vi "CSConnect.ProcCases.vi"(0 "i ref in":refnum<vi>, 1 "selector":string, 2 "Data":T1, 3 "call cluster":T2={"Object"="", "Selector"="", "CallType"=enum."synchronous", "Async Object"="", "Async Selector"="", "Data Descriptor"="", "Data"=[], "Error #"=0, "Expire"=0}, 5 "error in (no error)":errorcluster) -> (14 "i ref out":refnum<vi>, 17 "answer cluster":T2={"Object"="", "Selector"="", "CallType"=enum."synchronous", "Async Object"="", "Async Selector"="", "Data Descriptor"="", "Data"=[], "Error #"=0, "Expire"=0}, 19 "error out":errorcluster)   [LabVIEW 2014, in "CSConnect.lvlib"]
doc: "This method is called by a process from within the default case in the event loop. The methods of a class that are linked to events will be called from THIS method. Add your code here."
uses:
  CSConnect.lvlib
  CSCore/CSSystem/CoreDefs/CoreDefs.call_type.ctl
  CSCore/BaseProcess/BaseProcess.descriptor string definition.ctl
  CSCore/CSSystem/CoreDefs/CoreDefs.rawDataType.ctl
  CSCore/CSApplicationBaseClasses/PSChannelBase/PSChannelBase.directionType.ctl
  CSCore/CSApplicationBaseClasses/PSChannelBase/PSChannelBase.serviceType.ctl
  CSCore/CSSystem/CoreLib/CoreLib.string 2 byte array.vi
  CSCore/CSSystem/CoreLib/CoreLib.double 2 byte array.vi
  CSCore/CSSystem/CoreLib/CoreLib.byte array 2 double.vi
  CSCore/CSSystem/CoreLib/CoreLib.byte array 2 short.vi
  CSCore/CSSystem/CoreLib/CoreLib.byte array 2 int.vi
  CSCore/CSSystem/CoreLib/CoreLib.lvlib
  CSCore/BaseProcess/BaseProcess.lvlib
  CSCore/CSApplicationBaseClasses/PSChannelBase/PSChannelBase.lvlib
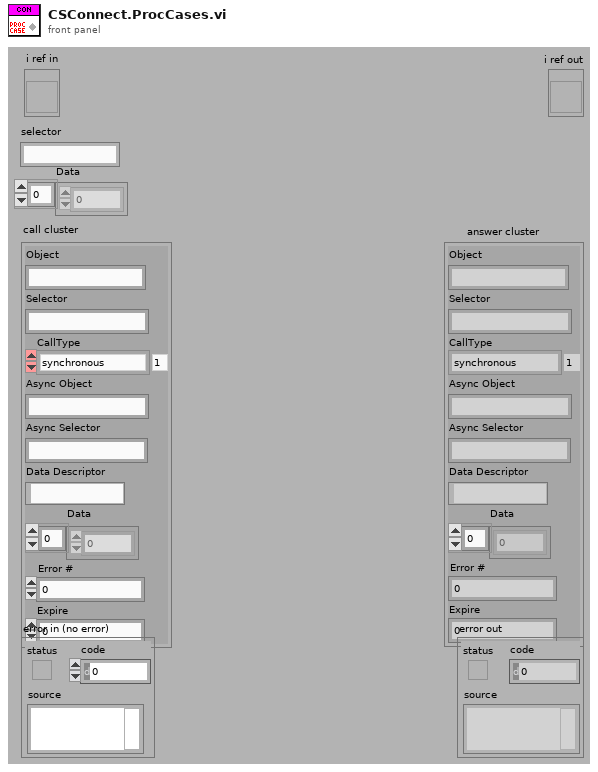
[diagram p1: front panel]
types:
  T1 = typedef "CoreDefs.rawDataType.ctl" = i8[]
  T2 = typedef "CoreDefs.call_type.ctl" = cluster{"Object":string, "Selector":string, "CallType":enum16{"simple", "synchronous", "asynchronous"}, "Async Object":string, "Async Selector":string, "Data Descriptor":T3, "Data":T1, "Error #":i32, "Expire":u32}
  T3 = typedef "BaseProcess.lvlib/BaseProcess.descriptor string definition.ctl" = string
  T4 = typedef "PSChannelBase.lvlib/PSChannelBase.serviceType.ctl" = enum16{"onOff", "voltage", "current", "tripCurrent", "rampUpSpeed", "rampDownSpeed", "status"}
  T5 = typedef "PSChannelBase.lvlib/PSChannelBase.directionType.ctl" = enum16{"unknown", "update actual value", "update nominal value", "update both"}
  T6 = typedef "CSConnect.lvlib/CSConnect.i attribute.ctl" = cluster{"In-Array":cluster{"Alias":string, "Value":dbl, "neededOuts":bool[]}[], "Out-Array":cluster{"ObjectName":string, "VoltFunctionName":string, "OnOffFunctionName":string, "Channel":string, "Calculation-Formula":string}[], "OutChannelsID":i32, "InOutMatrixID":i32}
  T7 = cluster{"ObjectName":string, "VoltFunctionName":string, "OnOffFunctionName":string, "Channel":string, "Calculation-Formula":string}[]
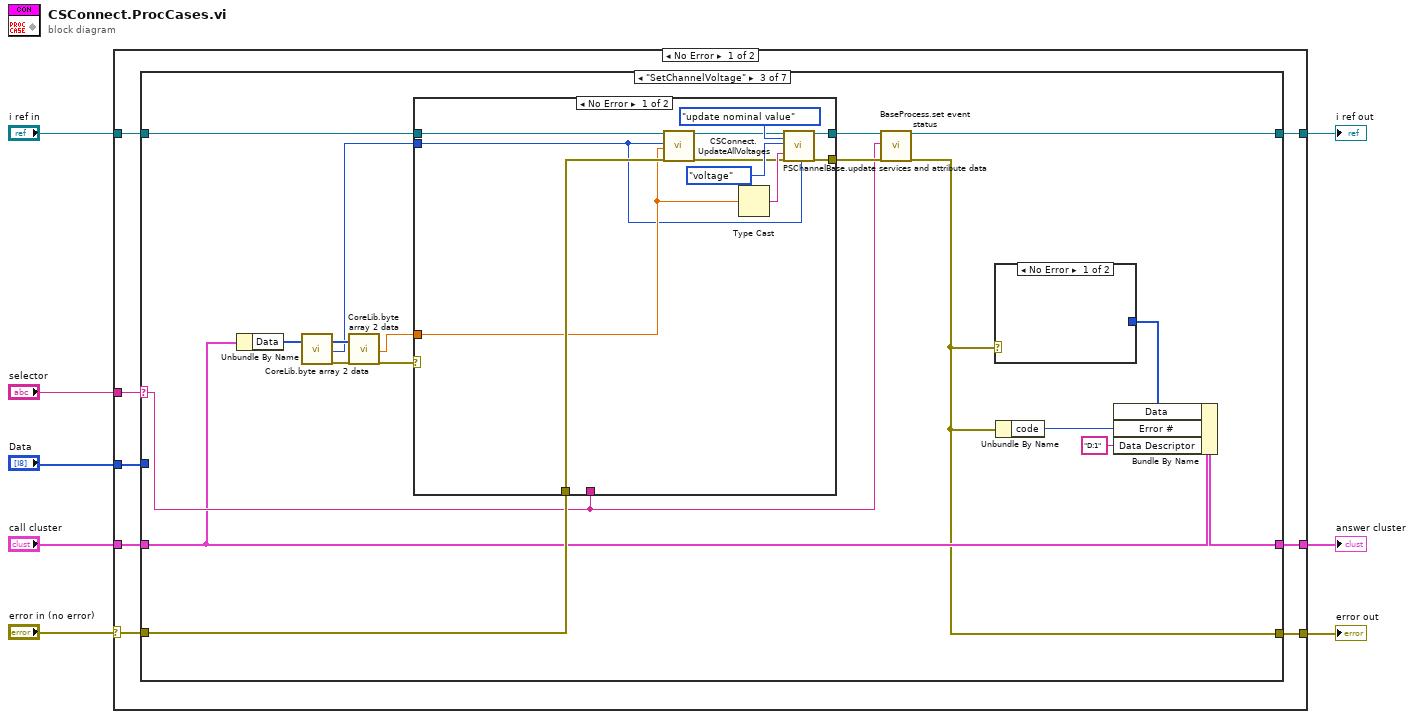
[diagram p0: block diagram]
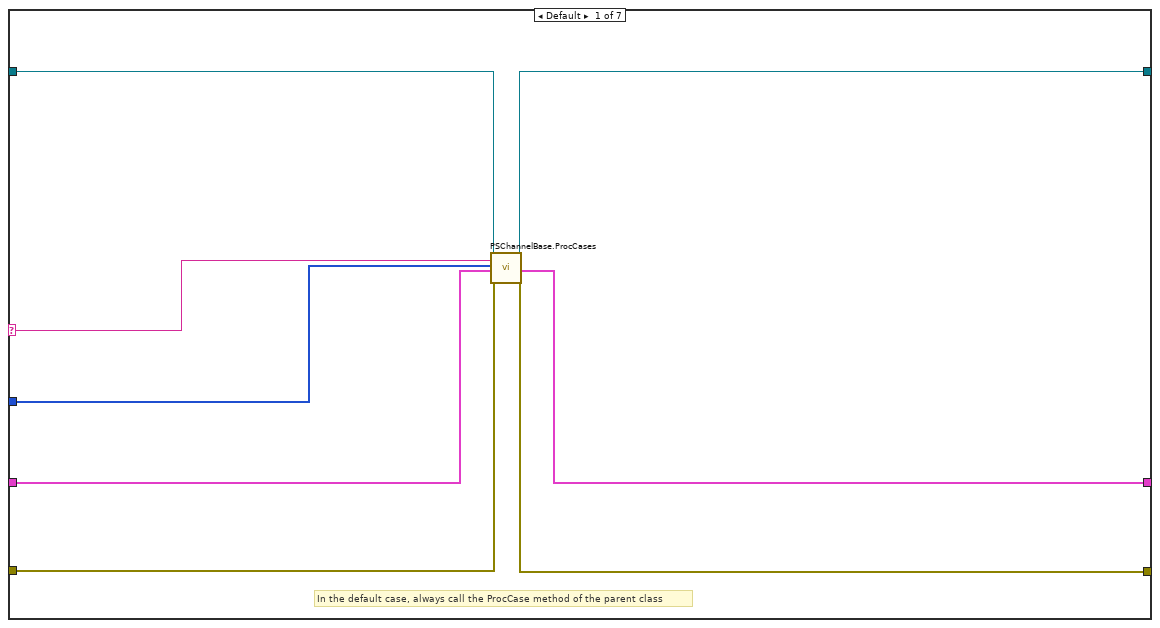
[diagram p2: hidden frame]
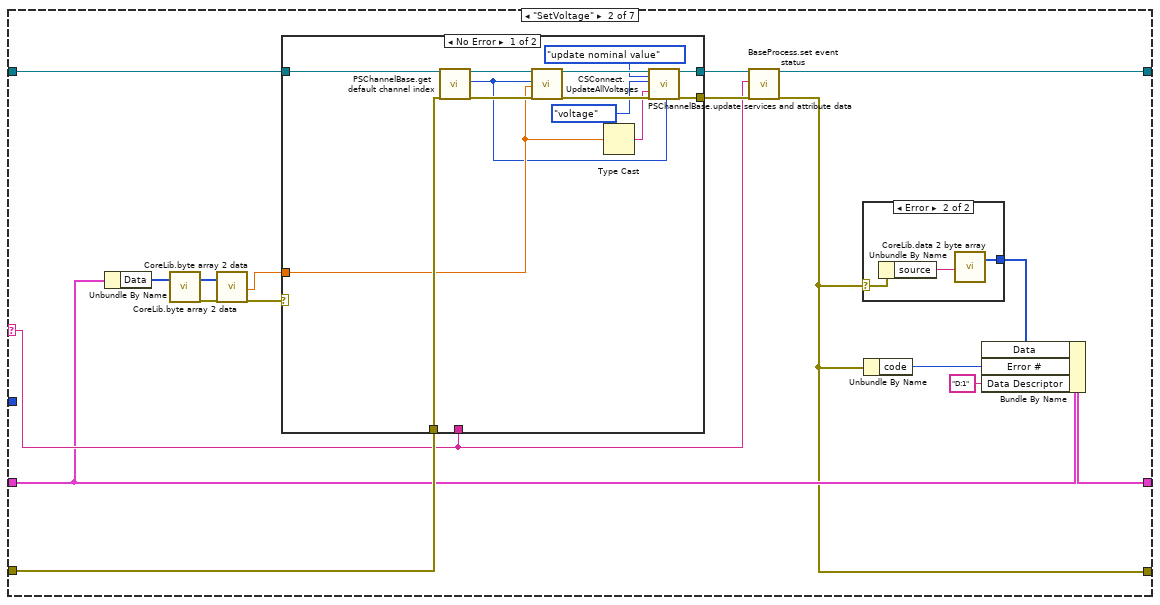
[diagram p3: hidden frame]
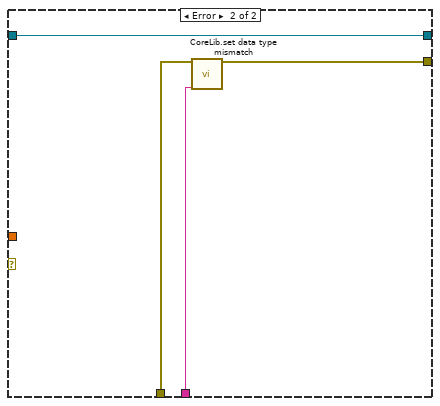
[diagram p5: hidden frame]
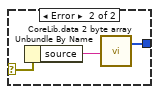
[diagram p6: hidden frame]
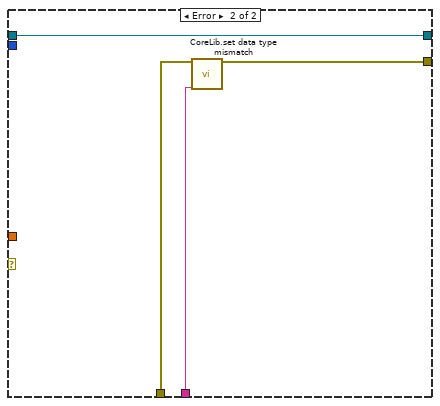
[diagram p7: hidden frame]
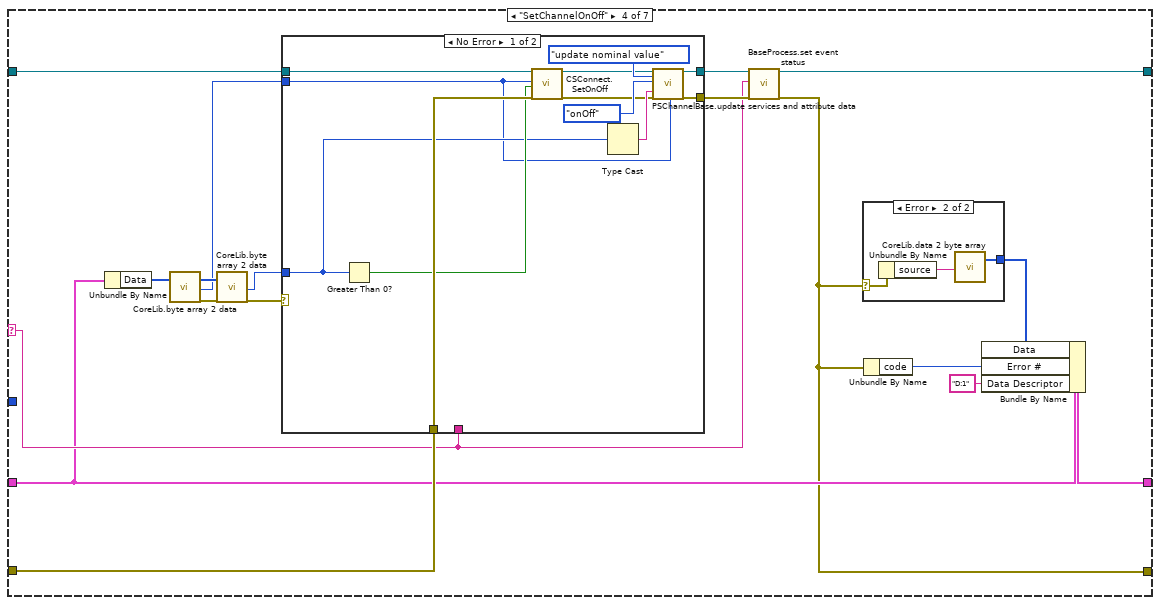
[diagram p8: hidden frame]
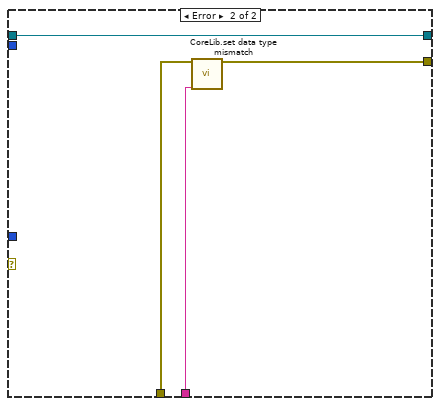
[diagram p10: hidden frame]
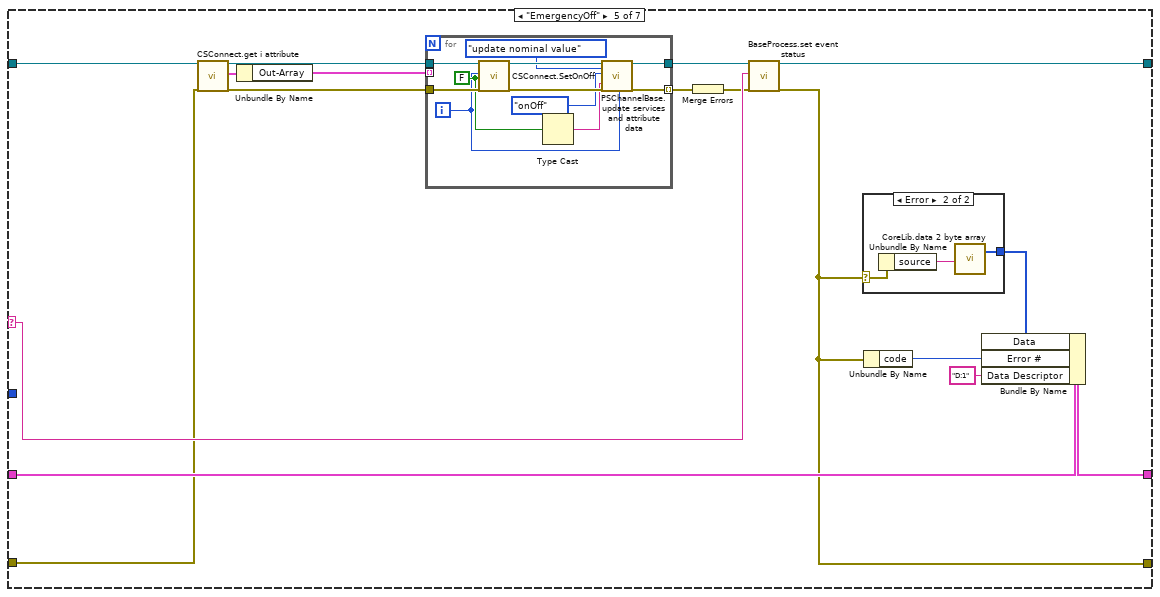
[diagram p11: hidden frame]
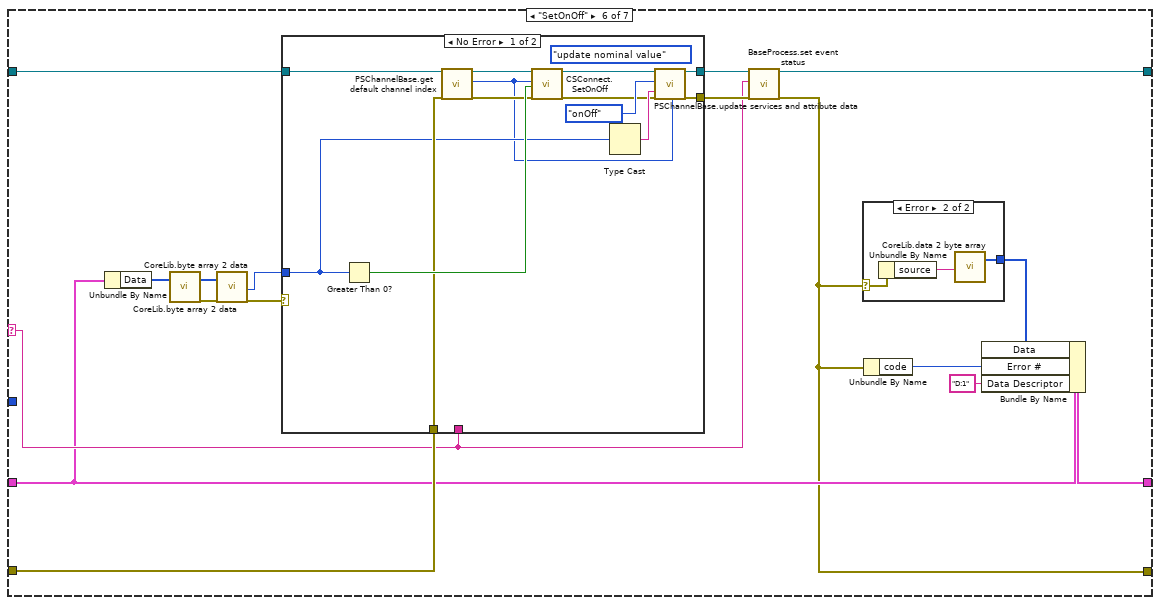
[diagram p13: hidden frame]
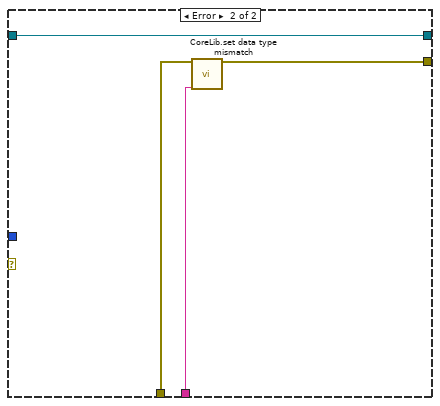
[diagram p15: hidden frame]
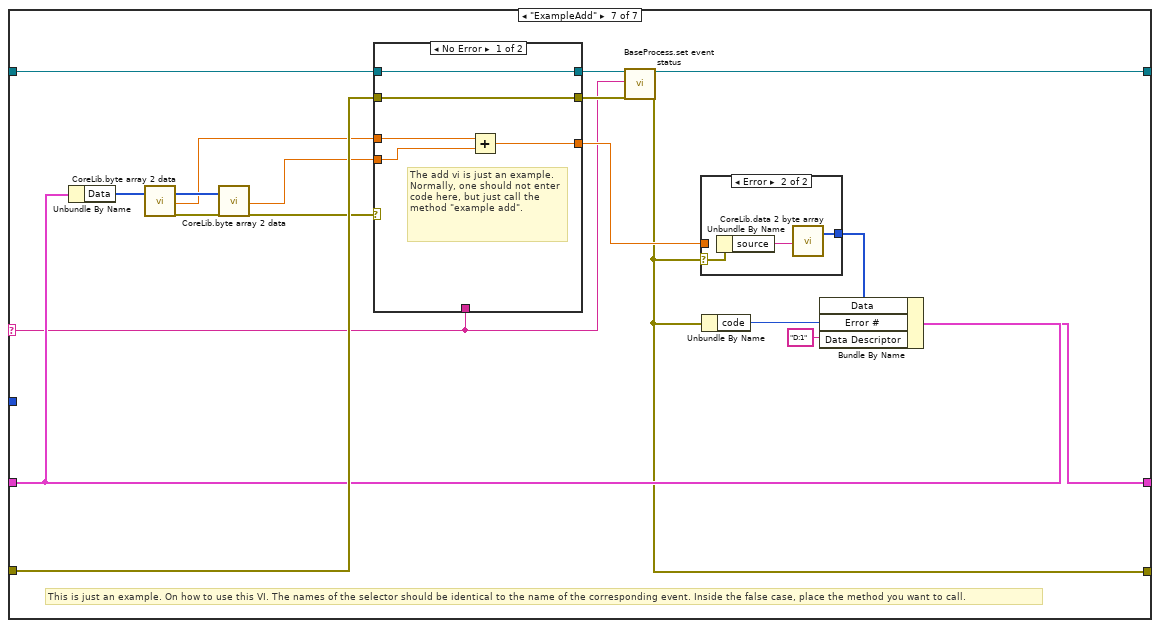
[diagram p16: hidden frame]
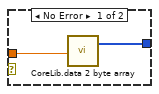
[diagram p17: hidden frame]
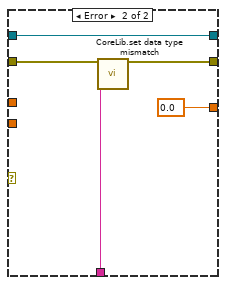
[diagram p18: hidden frame]
diagram:
  n1 = case shown="No Error" "error in (no error)" {
    selector: "error in (no error)" -> [w9 w237]
    tunnel: "selector" -> [w16 _]
    tunnel: [w15 w238] -> w7
    tunnel: "Data" -> [w14 _]
    tunnel: "call cluster" -> [w13 w238]
    tunnel: "i ref in" -> [w12 w239]
    tunnel: [w11 w239] -> w3
    tunnel: [w10 w237] -> w2
    frame No Error {
      n2 = case shown="\"SetChannelVoltage\"" w16 {
        selector: w16 -> [w19 w31 w69 w105 w148 w172 w211]
        tunnel: w14 -> [w17 _ _ _ _ _ _]
        tunnel: w12 -> [w18 w36 w74 w110 w141 w177 w221]
        tunnel: [w24 w33 w71 w107 w150 w174 w210] -> w11
        tunnel: w13 -> [w20 w27 w65 w101 w144 w168 w217]
        tunnel: [w21 w26 w64 w100 w143 w167 w216] -> w15
        tunnel: w9 -> [w23 w35 w73 w109 w139 w176 w220]
        tunnel: [w22 w25 w63 w99 w142 w166 w212] -> w10
        frame Default {
          # "In the default case, always call the ProcCase method of the parent class"
          n3 = call "PSChannelBase.ProcCases.vi"("i ref in"=w18, "selector"=w19, "Data"=w17, "call cluster"=w20, "error in (no error)"=w23) -> ("i ref out"=w24:refnum<vi>, "answer cluster"=w21:T2, "error out"=w22:errorcluster)  [unwired: 12 in]
        }
        frame "SetVoltage" {
          n4 = Unbundle By Name(w27) -> ("Data"=w41:T1)
          n5 = call-poly "CoreLib.byte array 2 data.vi"("byteArray"=w41) -> ("byteArray out"=w40:T1, "error out"=w39:errorcluster)  [unwired: 16 in, 1 out]
          n6 = call-poly "CoreLib.byte array 2 data.vi"("byteArray"=w40, "error in (no error)"=w39) -> ("d64"=w37:dbl, "error out"=w38:errorcluster)  [unwired: 15 in, 1 out]
          n7 = case shown="No Error" w38 {
            tunnel: w37 -> [w47 _]
            tunnel: w36 -> [w57 w61]
            tunnel: w35 -> [w54 w60]
            tunnel: [w52 w61] -> w34
            tunnel: [w50 w59] -> w32
            tunnel: w31 -> [_ w58]
            frame No Error {
              n8 = call "PSChannelBase.get default channel index.vi"("i ref in"=w57, "error in (no error)"=w54) -> ("i ref out"=w56:refnum<vi>, "defaultChannelIndex"=w45:i32, "error out"=w55:errorcluster)  [unwired: 15 in]
              n9 = call "CSConnect.UpdateAllVoltages.vi"("i ref in"=w56, "In-channel number"=w45, "In-Voltage"=w47, "error in (no error)"=w55) -> ("i ref out"=w53:refnum<vi>, "error out"=w51:errorcluster)  [unwired: 14 in]
              n10 = Type Cast(x=w47) -> (*(type *) &x=w48:string)  [unwired: 1 in]
              n11 = call "PSChannelBase.update services and attribute data.vi"("i ref in"=w53, "direction"=PSChannelBase.directionType."update nominal value", "service"=PSChannelBase.serviceType."voltage", "value"=w48, "error in (no error)"=w51, "channelNumber"=w45) -> ("i ref out"=w52:refnum<vi>, "error out"=w50:errorcluster)  [unwired: 11 in, 1 out]
            }
            frame Error {
              n12 = call "CoreLib.set data type mismatch.vi"("error in (no error)"=w60, "error source"=w58) -> ("error out"=w59:errorcluster)  [unwired: 17 in]
            }
          }
          n13 = call "BaseProcess.set event status.vi"("i ref in"=w34, "EventStatus"=w31, "error in (no error)"=w32) -> ("i ref out"=w33:refnum<vi>, "error out"=w25:errorcluster)  [unwired: 14 in, 1 out]
          n14 = case shown="Error" w25 {
            selector: w25 -> [_ w44]
            tunnel: [_ w43] -> w29
            frame No Error {
            }
            frame Error {
              n15 = Unbundle By Name(w44) -> ("source"=w42:string)
              n16 = call-poly "CoreLib.data 2 byte array.vi"("string"=w42) -> ("byteArray out"=w43:T1)  [unwired: 18 in]
            }
          }
          n17 = Unbundle By Name(w25) -> ("code"=w30:i32)
          n18 = Bundle By Name(cluster=w27, "Data"=w29, "Error #"=w30, "Data Descriptor"="D:1") -> (w26:T2)
        }
        frame "SetChannelVoltage" {
          n19 = Unbundle By Name(w65) -> ("Data"=w79:T1)
          n20 = call-poly "CoreLib.byte array 2 data.vi"("byteArray"=w79) -> ("byteArray out"=w78:T1, "i32"=w62:i32, "error out"=w77:errorcluster)  [unwired: 16 in]
          n21 = call-poly "CoreLib.byte array 2 data.vi"("byteArray"=w78, "error in (no error)"=w77) -> ("d64"=w75:dbl, "error out"=w76:errorcluster)  [unwired: 15 in, 1 out]
          n22 = case shown="No Error" w76 {
            tunnel: w75 -> [w86 _]
            tunnel: w74 -> [w93 w97]
            tunnel: w73 -> [w92 w96]
            tunnel: [w83 w97] -> w72
            tunnel: [w84 w95] -> w70
            tunnel: w69 -> [_ w94]
            tunnel: w62 -> [w85 _]
            frame No Error {
              n23 = call "CSConnect.UpdateAllVoltages.vi"("i ref in"=w93, "In-channel number"=w85, "In-Voltage"=w86, "error in (no error)"=w92) -> ("i ref out"=w88:refnum<vi>, "error out"=w87:errorcluster)  [unwired: 14 in]
              n24 = Type Cast(x=w86) -> (*(type *) &x=w90:string)  [unwired: 1 in]
              n25 = call "PSChannelBase.update services and attribute data.vi"("i ref in"=w88, "direction"=PSChannelBase.directionType."update nominal value", "service"=PSChannelBase.serviceType."voltage", "value"=w90, "error in (no error)"=w87, "channelNumber"=w85) -> ("i ref out"=w83:refnum<vi>, "error out"=w84:errorcluster)  [unwired: 11 in, 1 out]
            }
            frame Error {
              n26 = call "CoreLib.set data type mismatch.vi"("error in (no error)"=w96, "error source"=w94) -> ("error out"=w95:errorcluster)  [unwired: 17 in]
            }
          }
          n27 = call "BaseProcess.set event status.vi"("i ref in"=w72, "EventStatus"=w69, "error in (no error)"=w70) -> ("i ref out"=w71:refnum<vi>, "error out"=w63:errorcluster)  [unwired: 14 in, 1 out]
          n28 = case shown="No Error" w63 {
            selector: w63 -> [_ w82]
            tunnel: [_ w81] -> w67
            frame No Error {
            }
            frame Error {
              n29 = Unbundle By Name(w82) -> ("source"=w80:string)
              n30 = call-poly "CoreLib.data 2 byte array.vi"("string"=w80) -> ("byteArray out"=w81:T1)  [unwired: 18 in]
            }
          }
          n31 = Unbundle By Name(w63) -> ("code"=w68:i32)
          n32 = Bundle By Name(cluster=w65, "Data"=w67, "Error #"=w68, "Data Descriptor"="D:1") -> (w64:T2)
        }
        frame "SetChannelOnOff" {
          n33 = Unbundle By Name(w101) -> ("Data"=w115:T1)
          n34 = call-poly "CoreLib.byte array 2 data.vi"("byteArray"=w115) -> ("byteArray out"=w114:T1, "i32"=w98:i32, "error out"=w113:errorcluster)  [unwired: 16 in]
          n35 = call-poly "CoreLib.byte array 2 data.vi"("byteArray"=w114, "error in (no error)"=w113) -> ("i16"=w111:i16, "error out"=w112:errorcluster)  [unwired: 15 in, 1 out]
          n36 = case shown="No Error" w112 {
            tunnel: w111 -> [w120 _]
            tunnel: w110 -> [w130 w134]
            tunnel: w109 -> [w129 w133]
            tunnel: [w123 w134] -> w108
            tunnel: [w124 w132] -> w106
            tunnel: w105 -> [_ w131]
            tunnel: w98 -> [w119 _]
            frame No Error {
              n37 = Greater Than 0?(x=w120) -> (x > 0?=w128:bool)
              n38 = call "CSConnect.SetOnOff.vi"("i ref in"=w130, "In-channel number"=w119, "On?"=w128, "error in (no error)"=w129) -> ("i ref out"=w122:refnum<vi>, "error out"=w121:errorcluster)  [unwired: 14 in]
              n39 = Type Cast(x=w120) -> (*(type *) &x=w126:string)  [unwired: 1 in]
              n40 = call "PSChannelBase.update services and attribute data.vi"("i ref in"=w122, "direction"=PSChannelBase.directionType."update nominal value", "service"=PSChannelBase.serviceType."onOff", "value"=w126, "error in (no error)"=w121, "channelNumber"=w119) -> ("i ref out"=w123:refnum<vi>, "error out"=w124:errorcluster)  [unwired: 11 in, 1 out]
            }
            frame Error {
              n41 = call "CoreLib.set data type mismatch.vi"("error in (no error)"=w133, "error source"=w131) -> ("error out"=w132:errorcluster)  [unwired: 17 in]
            }
          }
          n42 = call "BaseProcess.set event status.vi"("i ref in"=w108, "EventStatus"=w105, "error in (no error)"=w106) -> ("i ref out"=w107:refnum<vi>, "error out"=w99:errorcluster)  [unwired: 14 in, 1 out]
          n43 = case shown="Error" w99 {
            selector: w99 -> [_ w118]
            tunnel: [_ w117] -> w103
            frame No Error {
            }
            frame Error {
              n44 = Unbundle By Name(w118) -> ("source"=w116:string)
              n45 = call-poly "CoreLib.data 2 byte array.vi"("string"=w116) -> ("byteArray out"=w117:T1)  [unwired: 18 in]
            }
          }
          n46 = Unbundle By Name(w99) -> ("code"=w104:i32)
          n47 = Bundle By Name(cluster=w101, "Data"=w103, "Error #"=w104, "Data Descriptor"="D:1") -> (w100:T2)
        }
        frame "EmergencyOff" {
          n48 = call "CSConnect.get i attribute.vi"("i ref in"=w141, "error in (no error)"=w139) -> ("i ref out"=w140:refnum<vi>, "i attribute"=w137:T6, "error out"=w138:errorcluster)  [unwired: 15 in]
          n49 = Unbundle By Name(w137) -> ("Out-Array"=w136:T7)
          n50 = for {
            tunnel: [w158] -> w151
            tunnel: [w159] -> w149 mode=indexing
            tunnel: w140 -> [w162]
            tunnel: w138 -> [w161]
            tunnel: w136 -> [_] mode=indexing
            i -> [w152]
            w153 = FALSE ("On?")
            n51 = call "CSConnect.SetOnOff.vi"("i ref in"=w162, "In-channel number"=w152, "On?"=w153, "error in (no error)"=w161) -> ("i ref out"=w157:refnum<vi>, "error out"=w160:errorcluster)  [unwired: 14 in]
            n52 = Type Cast(x=w153) -> (*(type *) &x=w154:string)  [unwired: 1 in]
            n53 = call "PSChannelBase.update services and attribute data.vi"("i ref in"=w157, "direction"=PSChannelBase.directionType."update nominal value", "service"=PSChannelBase.serviceType."onOff", "value"=w154, "error in (no error)"=w160, "channelNumber"=w152) -> ("i ref out"=w158:refnum<vi>, "error out"=w159:errorcluster)  [unwired: 11 in, 1 out]
          }
          n54 = Merge Errors(w149) -> (w135:errorcluster)
          n55 = call "BaseProcess.set event status.vi"("i ref in"=w151, "EventStatus"=w148, "error in (no error)"=w135) -> ("i ref out"=w150:refnum<vi>, "error out"=w142:errorcluster)  [unwired: 14 in, 1 out]
          n56 = case shown="Error" w142 {
            selector: w142 -> [_ w165]
            tunnel: [_ w164] -> w146
            frame No Error {
            }
            frame Error {
              n57 = Unbundle By Name(w165) -> ("source"=w163:string)
              n58 = call-poly "CoreLib.data 2 byte array.vi"("string"=w163) -> ("byteArray out"=w164:T1)  [unwired: 18 in]
            }
          }
          n59 = Unbundle By Name(w142) -> ("code"=w147:i32)
          n60 = Bundle By Name(cluster=w144, "Data"=w146, "Error #"=w147, "Data Descriptor"="D:1") -> (w143:T2)
        }
        frame "SetOnOff" {
          n61 = Unbundle By Name(w168) -> ("Data"=w182:T1)
          n62 = call-poly "CoreLib.byte array 2 data.vi"("byteArray"=w182) -> ("byteArray out"=w181:T1, "error out"=w180:errorcluster)  [unwired: 16 in, 1 out]
          n63 = call-poly "CoreLib.byte array 2 data.vi"("byteArray"=w181, "error in (no error)"=w180) -> ("i16"=w178:i16, "error out"=w179:errorcluster)  [unwired: 15 in, 1 out]
          n64 = case shown="No Error" w179 {
            tunnel: w178 -> [w187 _]
            tunnel: w177 -> [w195 w202]
            tunnel: w176 -> [w196 w201]
            tunnel: [w190 w202] -> w175
            tunnel: [w191 w200] -> w173
            tunnel: w172 -> [_ w199]
            frame No Error {
              (unwired) PSChannelBase.directionType."update nominal value" ("direction")
              n65 = Greater Than 0?(x=w187) -> (x > 0?=w198:bool)
              n66 = call "PSChannelBase.get default channel index.vi"("i ref in"=w195, "error in (no error)"=w196) -> ("i ref out"=w194:refnum<vi>, "defaultChannelIndex"=w186:i32, "error out"=w197:errorcluster)  [unwired: 15 in]
              n67 = call "CSConnect.SetOnOff.vi"("i ref in"=w194, "In-channel number"=w186, "On?"=w198, "error in (no error)"=w197) -> ("i ref out"=w189:refnum<vi>, "error out"=w188:errorcluster)  [unwired: 14 in]
              n68 = Type Cast(x=w187) -> (*(type *) &x=w193:string)  [unwired: 1 in]
              n69 = call "PSChannelBase.update services and attribute data.vi"("i ref in"=w189, "service"=PSChannelBase.serviceType."onOff", "value"=w193, "error in (no error)"=w188, "channelNumber"=w186) -> ("i ref out"=w190:refnum<vi>, "error out"=w191:errorcluster)  [unwired: 12 in, 1 out]
            }
            frame Error {
              n70 = call "CoreLib.set data type mismatch.vi"("error in (no error)"=w201, "error source"=w199) -> ("error out"=w200:errorcluster)  [unwired: 17 in]
            }
          }
          n71 = call "BaseProcess.set event status.vi"("i ref in"=w175, "EventStatus"=w172, "error in (no error)"=w173) -> ("i ref out"=w174:refnum<vi>, "error out"=w166:errorcluster)  [unwired: 14 in, 1 out]
          n72 = case shown="Error" w166 {
            selector: w166 -> [_ w185]
            tunnel: [_ w184] -> w170
            frame No Error {
            }
            frame Error {
              n73 = Unbundle By Name(w185) -> ("source"=w183:string)
              n74 = call-poly "CoreLib.data 2 byte array.vi"("string"=w183) -> ("byteArray out"=w184:T1)  [unwired: 18 in]
            }
          }
          n75 = Unbundle By Name(w166) -> ("code"=w171:i32)
          n76 = Bundle By Name(cluster=w168, "Data"=w170, "Error #"=w171, "Data Descriptor"="D:1") -> (w167:T2)
        }
        frame "ExampleAdd" {
          # "This is just an example. On how to use this VI. The names of the selector should be identical to the name of the corresponding event. Inside the false case, place the method you want to call."
          n77 = Unbundle By Name(w217) -> ("Data"=w208:T1)
          n78 = call-poly "CoreLib.byte array 2 data.vi"("byteArray"=w208) -> ("byteArray out"=w206:T1, "d64"=w204:dbl, "error out"=w207:errorcluster)  [unwired: 16 in]
          n79 = call-poly "CoreLib.byte array 2 data.vi"("byteArray"=w206, "error in (no error)"=w207) -> ("d64"=w203:dbl, "error out"=w205:errorcluster)  [unwired: 15 in, 1 out]
          n80 = case shown="No Error" w205 {
            tunnel: [w228 w236] -> w214
            tunnel: w221 -> [w228 w236]
            tunnel: w220 -> [w229 w235]
            tunnel: [w229 w234] -> w213
            tunnel: w203 -> [w231 _]
            tunnel: [w230 0.0] -> w219
            tunnel: w211 -> [_ w232]
            tunnel: w204 -> [w227 _]
            frame No Error {
              # "The add vi is just an example. Normally, one should not enter code here, but just call the method \"example add\"."
              n81 = Add(x=w227, y=w231) -> (x+y=w230:dbl)
            }
            frame Error {
              n82 = call "CoreLib.set data type mismatch.vi"("error in (no error)"=w235, "error source"=w232) -> ("error out"=w234:errorcluster)  [unwired: 17 in]
            }
          }
          n83 = call "BaseProcess.set event status.vi"("i ref in"=w214, "EventStatus"=w211, "error in (no error)"=w213) -> ("i ref out"=w210:refnum<vi>, "error out"=w212:errorcluster)  [unwired: 14 in, 1 out]
          n84 = case shown="Error" w212 {
            selector: w212 -> [_ w226]
            tunnel: [w222 w225] -> w215
            tunnel: w219 -> [w223 _]
            frame No Error {
              n85 = call-poly "CoreLib.data 2 byte array.vi"("f64"=w223) -> ("byteArray out"=w222:T1)  [unwired: 18 in]
            }
            frame Error {
              n86 = Unbundle By Name(w226) -> ("source"=w224:string)
              n87 = call-poly "CoreLib.data 2 byte array.vi"("string"=w224) -> ("byteArray out"=w225:T1)  [unwired: 18 in]
            }
          }
          n88 = Unbundle By Name(w212) -> ("code"=w218:i32)
          n89 = Bundle By Name(cluster=w217, "Data"=w215, "Error #"=w218, "Data Descriptor"="D:1") -> (w216:T2)
        }
      }
    }
    frame Error {
    }
  }
  "answer cluster" <- w7
  "i ref out" <- w3
  "error out" <- w2
